vi "Sparge_stop.vi"() -> ()   [LabVIEW 2021]
panel:
  out "Sparge_stop":bool
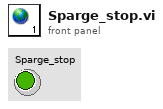
[diagram p1: front panel]
diagram:
